vi "append_to_disk.vi"(1 "write info file?":bool, 3 "time stamp":timestamp, 4 "File identifier":string, 5 "file info":string, 6 "Data":dbl[][](array[numeric])) -> (0 "error out":errorcluster, 2 "Path":path)   [LabVIEW 2012]
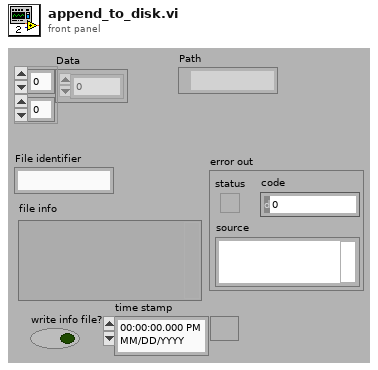
[diagram p1: front panel]
types:
  T1 = enum16{"open", "replace", "create", "open or create", "replace or create", "replace or create with confirmation"}
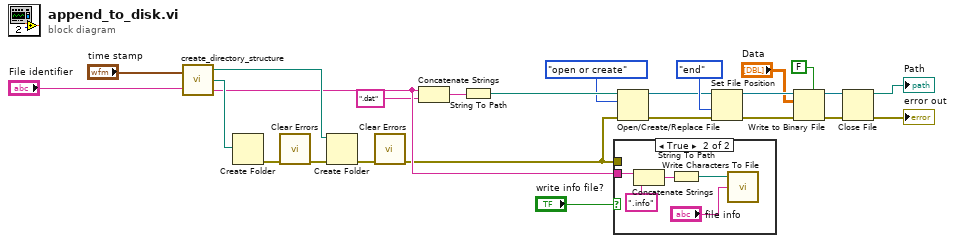
[diagram p0: block diagram]
diagram:
  n1 = call "create_directory_structure.vi"("time stamp"="time stamp", "File identifier"="File identifier") -> ("todays path"=w23:path, "Basepath"=w24:path, "filepath"=w22:string)
  n2 = Create Folder(path (use dialog)=w24) -> (error out=w3:errorcluster)  [unwired: 2 in, 2 out]
  n3 = call <vilib>:"Clear Errors.vi"("error in (no error)"=w3) -> ("error out"=w4:errorcluster)  [unwired: 6 in]
  n4 = Create Folder(path (use dialog)=w23, error in=w4) -> (error out=w2:errorcluster)  [unwired: 1 in, 2 out]
  n5 = call <vilib>:"Clear Errors.vi"("error in (no error)"=w2) -> ("error out"=w1:errorcluster)  [unwired: 6 in]
  n6 = Concatenate Strings(w22, ".dat" ("string")) -> (w5:string)
  n7 = String To Path(string=w5) -> (path=w16:path)
  n8 = case shown="True" "write info file?" {
    tunnel: w22 -> [_ w27]
    tunnel: w1 -> [_ _]
    frame False {
    }
    frame True {
      n9 = Concatenate Strings(w27, ".info" ("string")) -> (w29:string)
      n10 = String To Path(string=w29) -> (path=w30:path)
      n11 = call <vilib>:"Write Characters To File.vi"("character string"="file info", "file path (dialog if empty)"=w30) -> ()  [unwired: 3 in, 1 out]
    }
  }
  n12 = Open/Create/Replace File(file path (use dialog)=w16, error in=w1, operation (0:open)=T1."open or create") -> (refnum out=w14:refnum<file>, error out=w9:errorcluster)  [unwired: 3 in, 1 out]
  n13 = Set File Position(refnum=w14, from (0:start)=enum16{"start", "end", "current"}."end", error in=w9) -> (refnum out=w13:refnum<file>, error out=w10:errorcluster)  [unwired: 1 in]
  n14 = Write to Binary File(file (use dialog)=w13, data="Data", error in=w10, 5:FALSE ("prepend array or string size? (T)")) -> (refnum out=w11:refnum<file>, error out=w12:errorcluster)  [unwired: 2 in, 1 out]
  n15 = Close File(refnum=w11, error in=w12) -> (path=→"Path":path, error out=→"error out":errorcluster)
